vi "listbox.vi"() -> ()   [LabVIEW 2024]
panel:
  out "Listbox 2":i32[](listbox)
  out "Listbox":i32[](listbox)
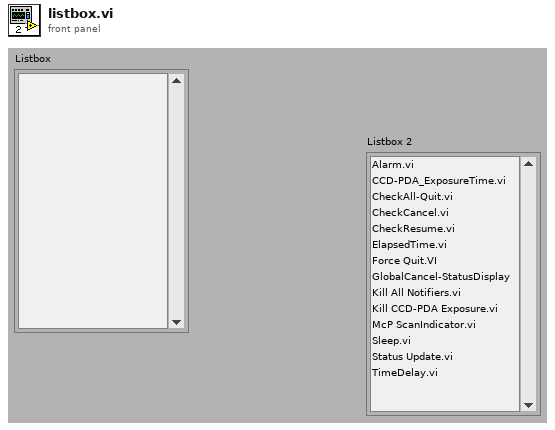
[diagram p1: front panel]
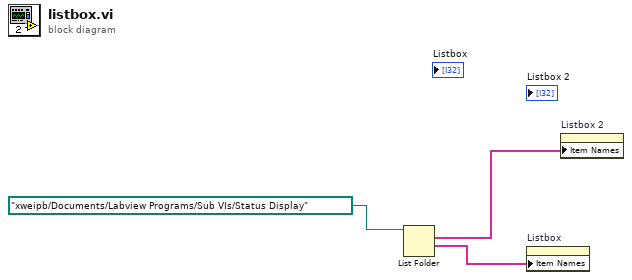
[diagram p0: block diagram]
diagram:
  n1 = List Folder(path=path "/xweipb/Documents/Labview Programs/Sub VIs/Status Display" ("directory path")) -> (filenames=w1:string[], folder names=w2:string[])  [unwired: 3 in, 2 out]
  n2 = property on="Listbox" class="LstBox (strict)"("Item Names"=w2) -> ()  [unwired: 2 in, 2 out]
  n3 = property on="Listbox 2" class="LstBox (strict)"("Item Names"=w1) -> ()  [unwired: 2 in, 2 out]
